vi "Get Params.vi"(1 "Point Correspondence Params in":refnum<class "Point Correspondence Params.lvclass">) -> (0 "Params":T1={"Refine"=TRUE, "Max Iterations"=0, "Inlier Threshold"=0.0})   [LabVIEW 2020, in "ar.lvlib" / "Point Correspondence Params.lvclass"]
doc: "Get Params."
uses:
  Point Correspondence Params.lvclass
  Params.ctl
  Point Correspondence Params.lvclass/Point Correspondence Params.ctl
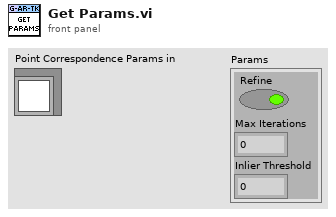
[diagram p1: front panel]
types:
  T1 = typedef "ar.lvlib/Point Correspondence Params.lvclass/Params.ctl" = cluster{"Refine":bool, "Max Iterations":i32, "Inlier Threshold":dbl}
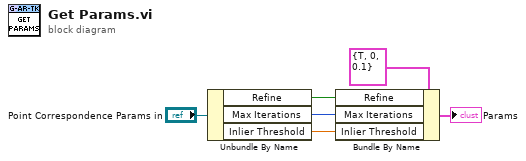
[diagram p0: block diagram]
diagram:
  n1 = Unbundle By Name("Point Correspondence Params in") -> ("Refine"=w4:bool, "Max Iterations"=w3:u16, "Inlier Threshold"=w2:dbl)
  n2 = Bundle By Name(cluster=T1 {"Refine"=TRUE, "Max Iterations"=0, "Inlier Threshold"=0.1} ("Params"), "Refine"=w4, "Max Iterations"=w3, "Inlier Threshold"=w2) -> (→"Params":T1)
